vi "CreateAi.vi"(0 "AI in":refnum<class "AI.lvclass">, 5 "error in (no error)":errorcluster, 11 "Scale":refnum<class "Scale_PiecedLinear.lvclass">, 12 "Tags":T1, 13 "Logger":refnum<class "Logger.lvclass">) -> (14 "AI out":refnum<class "AI.lvclass">, 19 "error out":errorcluster)   [LabVIEW 2019, in "AI.lvclass"]
uses:
  AI.lvclass
  C:/Users/ANENKOV_V1/Desktop/src/Signal_class/Signal.lvclass
  Proccess_class/TAGs.ctl
  Logger_class/Logger.lvclass
  PiecedLinearScale_class/Scale_PiecedLinear.lvclass
  AI.lvclass/AI.ctl
  TypeDef/AlarmType.ctl
  Signal_class/Signal.lvclass
  AnalogComparator_class/AnalogComparator.lvclass
  Proccess_class/Proccess.lvclass
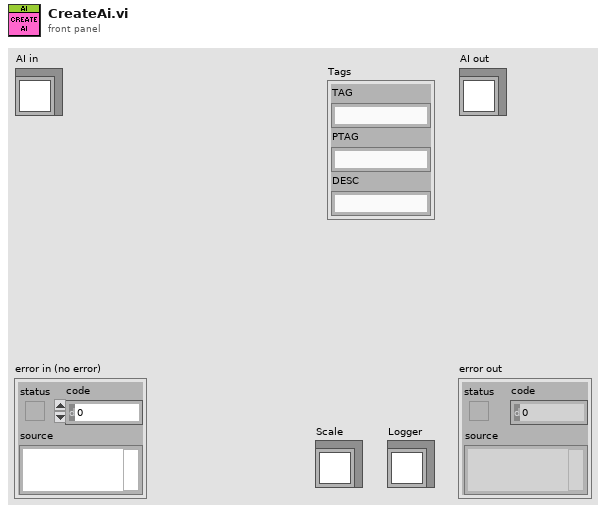
[diagram p1: front panel]
types:
  T1 = typedef "Proccess.lvclass/TAGs.ctl" = cluster{"TAG":string, "PTAG":string, "DESC":string}
  T2 = typedef "AlarmType.ctl" = enum16{"Normal", "Warning", "Alarm"}
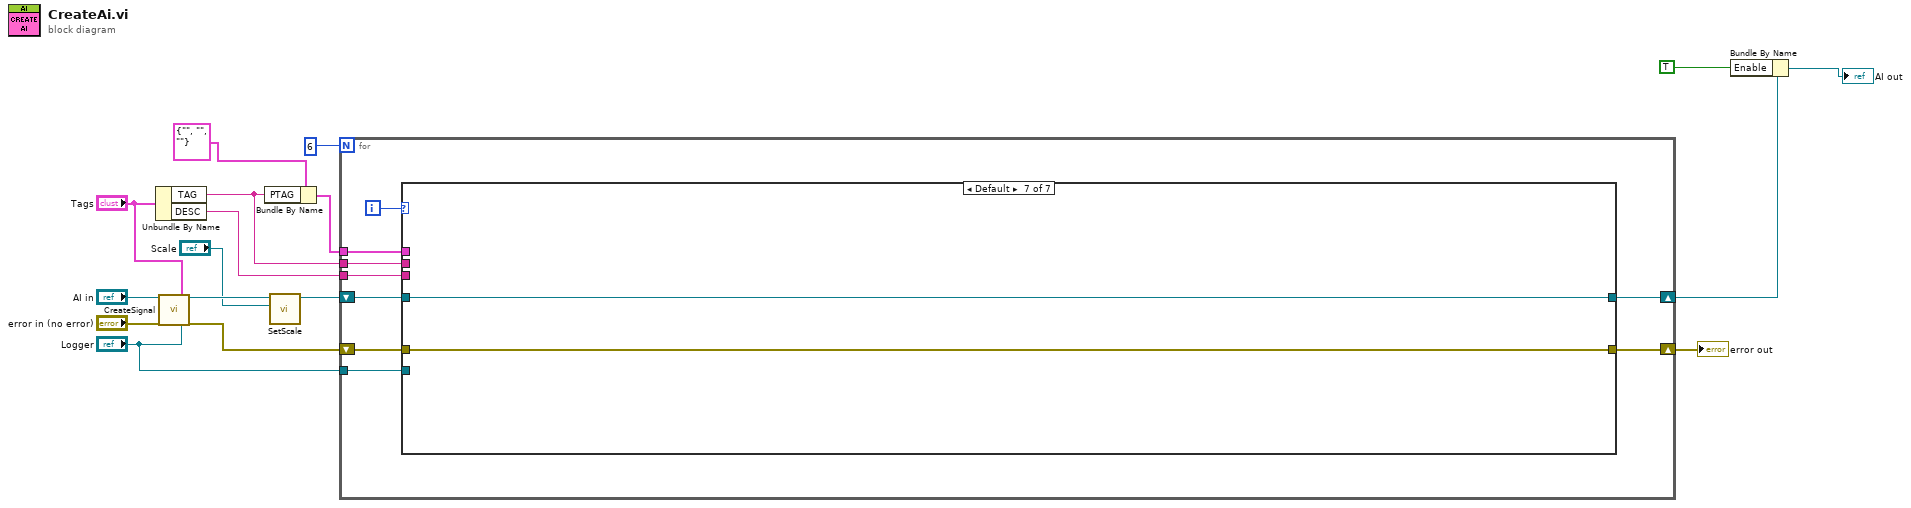
[diagram p0: block diagram]
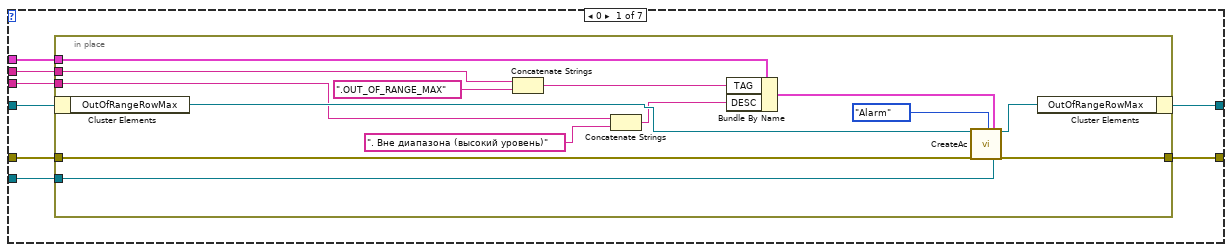
[diagram p2: hidden frame]
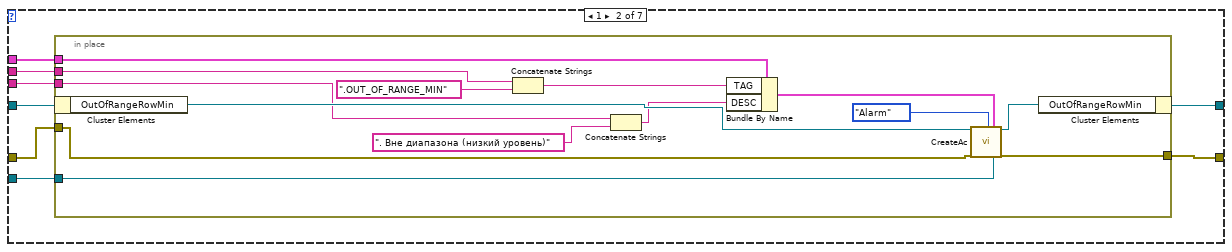
[diagram p3: hidden frame]
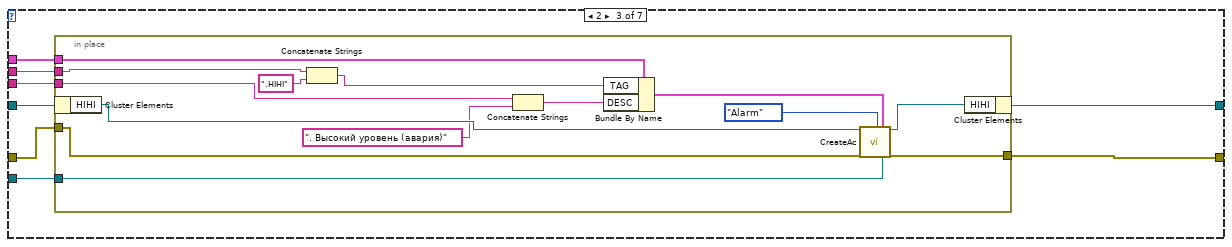
[diagram p4: hidden frame]
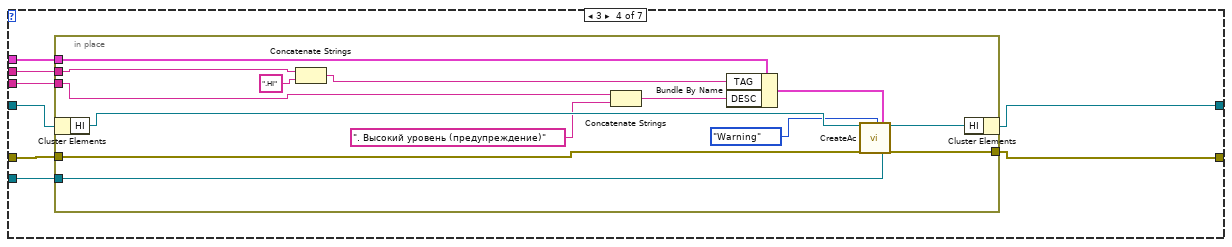
[diagram p5: hidden frame]
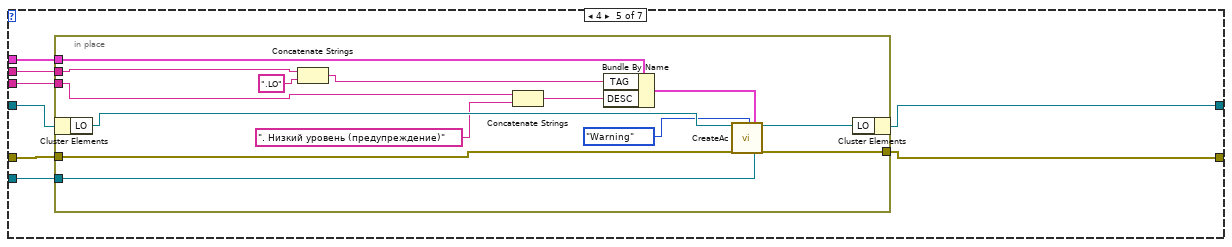
[diagram p6: hidden frame]
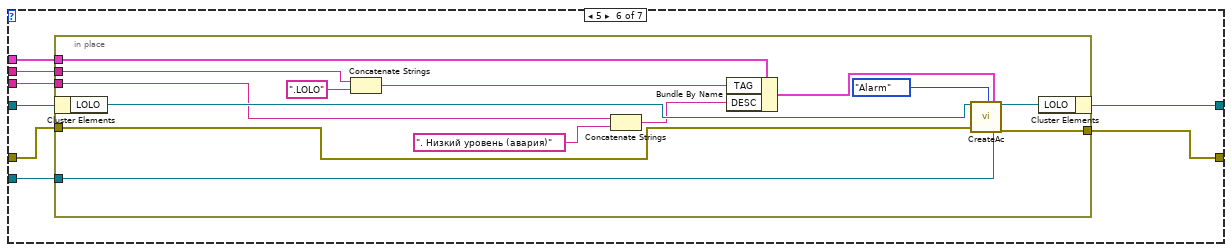
[diagram p7: hidden frame]
diagram:
  n1 = Unbundle By Name("Tags") -> ("TAG"=w8:string, "DESC"=w3:string)
  n2 = call "CreateSignal.vi"("Signal in"="AI in", "error in (no error)"="error in (no error)", "Tags"="Tags", "Logger"="Logger") -> ("Signal out"=w15:refnum<class "AI.lvclass">, "error out"=w6:errorcluster)  [unwired: 14 in]
  n3 = Bundle By Name(cluster=T1 {"TAG"="", "PTAG"="", "DESC"=""} ("Tags"), "PTAG"=w8) -> (w9:T1)
  n4 = call "SetScale.vi"("Scale"="Scale", "Sig_AI in"=w15) -> ("Sig_AI out"=w13:refnum<class "AI.lvclass">)  [unwired: 9 in]
  n5 = for {
    N: 6 -> [_]
    tunnel: w9 -> [w24]
    tunnel: w8 -> [w23]
    shift-right: [w25] -> w12
    shift-left: w13 -> [w26]
    shift-right: [w21] -> w5
    shift-left: w6 -> [w22]
    tunnel: "Logger" -> [w19]
    tunnel: w3 -> [w18]
    i -> [w20]
    n6 = case shown="Default" w20 {
      tunnel: w26 -> [w34 w56 w78 w100 w122 w144 w160]
      tunnel: [w33 w55 w77 w99 w121 w143 w160] -> w25
      tunnel: w24 -> [w32 w54 w76 w98 w120 w142 _]
      tunnel: w23 -> [w31 w53 w75 w97 w119 w141 _]
      tunnel: w22 -> [w30 w52 w74 w96 w118 w140 w159]
      tunnel: [w29 w51 w73 w95 w117 w139 w159] -> w21
      tunnel: w19 -> [w28 w50 w72 w94 w116 w138 _]
      tunnel: w18 -> [w27 w49 w71 w93 w115 w137 _]
      frame 0 {
        n7 = in-place {
          in-place-border: w32 -> [w46]
          in-place-border: w31 -> [w44]
          in-place-border: w30 -> [w41]
          in-place-border: [w40] -> w29
          in-place-border: w28 -> [w39]
          in-place-border: w27 -> [w36]
          n8 = in-place-cluster #1(w34) -> ("OutOfRangeRowMax"=w48:refnum<class "AnalogComparator.lvclass">)
          n9 = Concatenate Strings(w44, ".OUT_OF_RANGE_MAX" ("string")) -> (w42:string)
          n10 = Concatenate Strings(w36, ". Вне диапазона (высокий уровень)" ("string")) -> (w35:string)
          n11 = Bundle By Name(cluster=w46, "TAG"=w42, "DESC"=w35) -> (w45:T1)
          n12 = call "CreateAc.vi"("AnalogComparator"=w48, "error in (no error)"=w41, "AlarmType"=AlarmType."Alarm", "Tags"=w45, "Logger"=w39) -> ("AnalogComparator out"=w47:refnum<class "AnalogComparator.lvclass">, "error out"=w40:errorcluster)  [unwired: 13 in]
          n13 = in-place-cluster #1("OutOfRangeRowMax"=w47) -> (w33:refnum<class "AI.lvclass">)
        }
      }
      frame 1 {
        n14 = in-place {
          in-place-border: w54 -> [w68]
          in-place-border: w53 -> [w66]
          in-place-border: w52 -> [w63]
          in-place-border: [w62] -> w51
          in-place-border: w50 -> [w61]
          in-place-border: w49 -> [w58]
          n15 = in-place-cluster #2(w56) -> ("OutOfRangeRowMin"=w70:refnum<class "AnalogComparator.lvclass">)
          n16 = Concatenate Strings(w66, ".OUT_OF_RANGE_MIN" ("string")) -> (w64:string)
          n17 = Concatenate Strings(w58, ". Вне диапазона (низкий уровень)" ("string")) -> (w57:string)
          n18 = Bundle By Name(cluster=w68, "TAG"=w64, "DESC"=w57) -> (w67:T1)
          n19 = call "CreateAc.vi"("AnalogComparator"=w70, "error in (no error)"=w63, "AlarmType"=AlarmType."Alarm", "Tags"=w67, "Logger"=w61) -> ("AnalogComparator out"=w69:refnum<class "AnalogComparator.lvclass">, "error out"=w62:errorcluster)  [unwired: 13 in]
          n20 = in-place-cluster #2("OutOfRangeRowMin"=w69) -> (w55:refnum<class "AI.lvclass">)
        }
      }
      frame 2 {
        n21 = in-place {
          in-place-border: w76 -> [w90]
          in-place-border: w75 -> [w88]
          in-place-border: w74 -> [w85]
          in-place-border: [w84] -> w73
          in-place-border: w72 -> [w83]
          in-place-border: w71 -> [w80]
          n22 = in-place-cluster #3(w78) -> ("HIHI"=w92:refnum<class "AnalogComparator.lvclass">)
          n23 = Concatenate Strings(w88, ".HIHI" ("string")) -> (w86:string)
          n24 = Concatenate Strings(w80, ". Высокий уровень (авария)" ("string")) -> (w79:string)
          n25 = Bundle By Name(cluster=w90, "TAG"=w86, "DESC"=w79) -> (w89:T1)
          n26 = call "CreateAc.vi"("AnalogComparator"=w92, "error in (no error)"=w85, "AlarmType"=AlarmType."Alarm", "Tags"=w89, "Logger"=w83) -> ("AnalogComparator out"=w91:refnum<class "AnalogComparator.lvclass">, "error out"=w84:errorcluster)  [unwired: 13 in]
          n27 = in-place-cluster #3("HIHI"=w91) -> (w77:refnum<class "AI.lvclass">)
        }
      }
      frame 3 {
        n28 = in-place {
          in-place-border: w98 -> [w112]
          in-place-border: w97 -> [w110]
          in-place-border: w96 -> [w108]
          in-place-border: [w107] -> w95
          in-place-border: w94 -> [w106]
          in-place-border: w93 -> [w102]
          n29 = in-place-cluster #4(w100) -> ("HI"=w114:refnum<class "AnalogComparator.lvclass">)
          n30 = Concatenate Strings(w110, ".HI" ("string")) -> (w103:string)
          n31 = Concatenate Strings(w102, ". Высокий уровень (предупреждение)" ("string")) -> (w101:string)
          n32 = Bundle By Name(cluster=w112, "TAG"=w103, "DESC"=w101) -> (w111:T1)
          n33 = call "CreateAc.vi"("AnalogComparator"=w114, "error in (no error)"=w108, "AlarmType"=AlarmType."Warning", "Tags"=w111, "Logger"=w106) -> ("AnalogComparator out"=w113:refnum<class "AnalogComparator.lvclass">, "error out"=w107:errorcluster)  [unwired: 13 in]
          n34 = in-place-cluster #4("HI"=w113) -> (w99:refnum<class "AI.lvclass">)
        }
      }
      frame 4 {
        n35 = in-place {
          in-place-border: w120 -> [w134]
          in-place-border: w119 -> [w132]
          in-place-border: w118 -> [w129]
          in-place-border: [w128] -> w117
          in-place-border: w116 -> [w127]
          in-place-border: w115 -> [w124]
          n36 = in-place-cluster #5(w122) -> ("LO"=w136:refnum<class "AnalogComparator.lvclass">)
          n37 = Concatenate Strings(w132, ".LO" ("string")) -> (w130:string)
          n38 = Concatenate Strings(w124, ". Низкий уровень (предупреждение)" ("string")) -> (w123:string)
          n39 = Bundle By Name(cluster=w134, "TAG"=w130, "DESC"=w123) -> (w133:T1)
          n40 = call "CreateAc.vi"("AnalogComparator"=w136, "error in (no error)"=w129, "AlarmType"=AlarmType."Warning", "Tags"=w133, "Logger"=w127) -> ("AnalogComparator out"=w135:refnum<class "AnalogComparator.lvclass">, "error out"=w128:errorcluster)  [unwired: 13 in]
          n41 = in-place-cluster #5("LO"=w135) -> (w121:refnum<class "AI.lvclass">)
        }
      }
      frame 5 {
        n42 = in-place {
          in-place-border: w142 -> [w156]
          in-place-border: w141 -> [w154]
          in-place-border: w140 -> [w151]
          in-place-border: [w150] -> w139
          in-place-border: w138 -> [w149]
          in-place-border: w137 -> [w145]
          n43 = in-place-cluster #6(w144) -> ("LOLO"=w158:refnum<class "AnalogComparator.lvclass">)
          n44 = Concatenate Strings(w154, ".LOLO" ("string")) -> (w152:string)
          n45 = Concatenate Strings(w145, ". Низкий уровень (авария)" ("string")) -> (w146:string)
          n46 = Bundle By Name(cluster=w156, "TAG"=w152, "DESC"=w146) -> (w155:T1)
          n47 = call "CreateAc.vi"("AnalogComparator"=w158, "error in (no error)"=w151, "AlarmType"=AlarmType."Alarm", "Tags"=w155, "Logger"=w149) -> ("AnalogComparator out"=w157:refnum<class "AnalogComparator.lvclass">, "error out"=w150:errorcluster)  [unwired: 13 in]
          n48 = in-place-cluster #6("LOLO"=w157) -> (w143:refnum<class "AI.lvclass">)
        }
      }
      frame Default {
      }
    }
  }
  "error out" <- w5
  n49 = Bundle By Name(cluster=w12, "Enable"=TRUE) -> (→"AI out":refnum<class "AI.lvclass">)
